vi "MDPtrMgr Sync.vi"(6 "timeout(10s)":u32=10, 8 "error in (no error)":errorcluster) -> (0 "error out":errorcluster, 1 "timeout?":bool, 4 "time esliped?":dbl)   [LabVIEW 2017, in "MDPtr.lvlib"]
uses:
  MDPtr.lvlib
  _MDPtrMgr/MDPtrMgr.lvclass
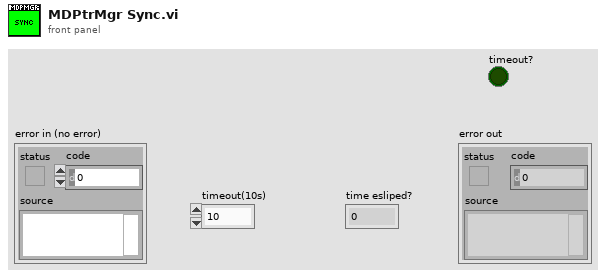
[diagram p1: front panel]
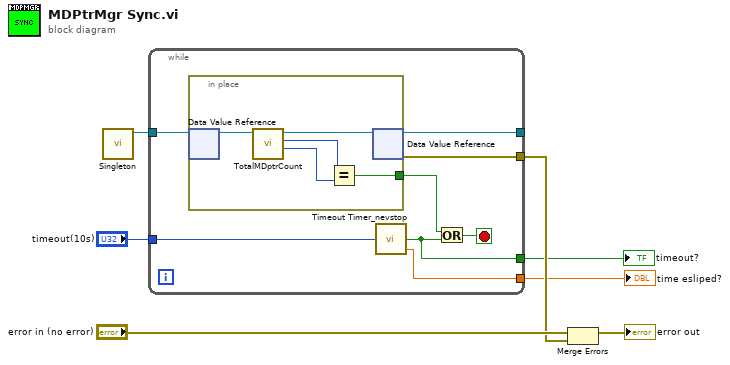
[diagram p0: block diagram]
diagram:
  n1 = call "Singleton.vi"() -> ("MDPtrMgrDVR"=w2:refnum<data-value>)  [unwired: 9 in, 2 out]
  n2 = while {
    tunnel: w2 -> [w15]
    tunnel: [w14] -> w5
    tunnel: "timeout(10s)" -> [w13]
    tunnel: [w10] -> w3
    tunnel: [w9] -> _
    tunnel: [w8] -> w1
    stop <- w11 stop-if-true
    n3 = in-place {
      in-place-border: [w16] -> w12
      n4 = in-place-dvr #1(w15) -> (w20:refnum<class "MDPtrMgr.lvclass">)  [unwired: 1 out]
      n5 = call "TotalMDptrCount.vi"("MDPtrMgr in"=w20) -> ("# free elements in queue"=w17:i32, "# elements in queue"=w18:i32, "MDPtrMgr out"=w19:refnum<class "MDPtrMgr.lvclass">)  [unwired: 6 in, 2 out]
      n6 = Equal?(x=w18, y=w17) -> (x = y?=w16:bool)
      n7 = in-place-dvr #1(w19) -> (w9:refnum<data-value>, w14:errorcluster)
    }
    n8 = call <userlib>:"Timeout Timer_nevstop.vi"("timeout(s)"=w13) -> ("timeout?"=w10:bool, "time esliped?"=w8:dbl)  [unwired: 7 in]
    n9 = Or(x=w12, y=w10) -> (x .or. y?=w11:bool)
  }
  "timeout?" <- w3
  "time esliped?" <- w1
  n10 = Merge Errors("error in (no error)", w5) -> (→"error out":errorcluster)
